vi "Destroy Message Queue Reference.vi"(8 "error in (no error)":errorcluster) -> (0 "error out":errorcluster)   [LabVIEW 2021, in "dcvmMessageQueue.lvlib"]
uses:
  dcvmMessageQueue.lvlib
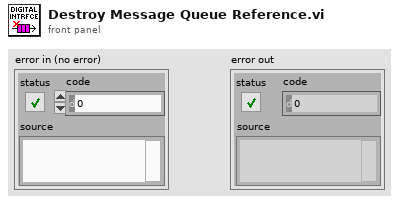
[diagram p1: front panel]
types:
  T1 = typedef "dcvmMessageQueue.lvlib/Message Queues.ctl" = cluster{"gRPC engine":refnum<queue>, "Digital engine":refnum<queue>}
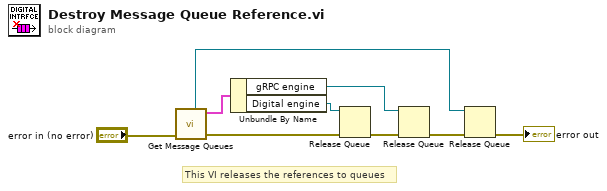
[diagram p0: block diagram]
diagram:
  # "This VI releases the references to queues"
  n1 = call "Get Message Queues.vi"("error in (no error)"="error in (no error)") -> ("error out"=w6:errorcluster, "AllMsgQueues QueueRef"=w8:T1, "MsgQueues QueueRef"=w1:refnum<queue>)  [unwired: 8 in]
  n2 = Unbundle By Name(w8) -> ("gRPC engine"=w5:refnum<queue>, "Digital engine"=w7:refnum<queue>)
  n3 = Release Queue(queue=w7, error in (no error)=w6) -> (error out=w4:errorcluster)  [unwired: 1 in, 2 out]
  n4 = Release Queue(queue=w5, error in (no error)=w4) -> (error out=w3:errorcluster)  [unwired: 1 in, 2 out]
  n5 = Release Queue(queue=w1, error in (no error)=w3) -> (error out=→"error out":errorcluster)  [unwired: 1 in, 2 out]
